vi "BMME385Project2_AmeenZafiruddin.vi"() -> ()   [LabVIEW 2022 SP3]
doc: "Read one the value of one analog channel from a LINX device."
uses:
  <vilib>/Analysis/3filter.llb/Filter Passband Type.ctl
  <vilib>/MakerHub/LINX/Public/Peripherals/Analog/Analog Read 1 Chan.vi
  <vilib>/MakerHub/LINX/Public/Peripherals/Digital/Digital Write N Chans.vi
  <vilib>/MakerHub/LINX/Public/Peripherals/Analog/Analog Read N Chans.vi
  <vilib>/MakerHub/LINX/Private/Local IO/LinxDigitalWrite.vi
  <vilib>/MakerHub/LINX/Public/Utilities/Check Channel.vi
  <vilib>/MakerHub/LINX/Private/Local IO/LinxAnalogRead.vi
  <vilib>/MakerHub/LINX/Private/Utilties/Generate Error.vi
  <vilib>/MakerHub/LINX/LMH-LINX.lvlib
  <vilib>/ptbypt/NI_PtbyPt.lvlib
  <vilib>/Analysis/NI_AAL_SigProc.lvlib
  <vilib>/Analysis/NI_AALBase.lvlib
panel:
  out "Diastolic Pressure":dbl
  out "Closest D Time":dbl
  out "Closest D Time Index":i32
  out "D Time":dbl
  out "D Location":dbl
  out "Systolic Pressure":dbl
  out "Closest S Time":dbl
  out "Closest S Time Index":i32
  out "S Time":dbl
  out "S Location":dbl
  out "Closest D Peak":dbl
  out "Closest D Peak Index":i32
  out "Closest S Peak":dbl
  out "Closest S Peak Index":i32
  out "Diastolic Peak Amp":dbl
  out "Systolic Peak Amp":dbl
  out "Mean Arterial Pressure (MAP)":dbl
  out "Closest MAP Time":dbl
  out "Closest MAP Index":i32
  out "MAP Time":dbl
  out "MAP Location":dbl
  out "MAP Peak Amp":dbl
  out "Amplitudes (mmHg)":dbl[](array[numeric])
  out "Locations":dbl[](array[numeric])
  in  "Peak Detection Threshold":dbl format="%0.2f"
  out "T Subset":dbl[](array[numeric])
  out "O Subset":dbl[](array[numeric])
  out "Oscillations (Bandpass Data) Subset":cluster{dbl[], dbl[]}[](graph)
  in  "Initialize\nFilter":bool
  in  "Filter Type":T1
  in  "Low Cutoff Frequency (Hz)":dbl=0.125 format="%0.3f"
  in  "High Cutoff Frequency (Hz)":dbl=0.45000000000000007 format="%0.3f"
  out "Oscillations (Bandpass Data) (mmHg)":dbl[](array[numeric])
  in  "Subset Start/Stop":bool
  out "Pressure (Raw Data) Subset":cluster{dbl[], dbl[]}[](graph)
  out "P Subset":dbl[](array[numeric])
  out "Time (s)":dbl[](array[numeric])
  out "Pressure (Raw Data) (mmHg)":dbl[](array[numeric])
  out "Pressure (Raw Data) (mmHg)":dbl(graph)
  in  "Digital Out (Gain)":bool[](array[boolean])
  in  "Digital Out Channels":u8[](array[numeric])=[10, 11, 12, 13]
  in  "Set Gain":bool
  in  "AI Channel":u8
  out "Loop Rate (Hz)":u32
  in  "Stop Button":bool
  out "Oscillations (Bandpass Data) (mmHg)":dbl(graph)
  in  "Serial Port":refnum<visa-resource-name>
  # "LINX Device Settings"
  # "Gain Settings"
  # "Filter Settings"
  # "HOW TO USE\n\n1. Connect appropriate hardware to computer via USB (Arduino + LTC615 + Pressure Transducer + BP Cuff)\n2. Select the COM Port (connected USB port) and Analog Channel (A0 - A1 on Arduino) under LINX Device Settings\n3. Set Gain via binary according to the appropriate digital channels (0001 = 128 Gain provided full range) under Gain Settings\n4. Set Filter to bandpass with a frequency range of 1 to 10 Hz under Filter Settings\n5. Click the Run Arrow\n6. Wrap the BP cuff around the patient and click the Initialize Filter button under Filter Settings\n7. Test to see if the raw and filtered pressure data are reading appropriately relative to the gauge attached to the BP cuff\n8. Pump up the cuff to 160 mmHg and begin to slowly release air\n9. Once the pressure reaches 140 mmHg, click the Subset Start/Stop button with an appropriate Peak Detection Threshold\n10. Continue to allow the air to release. Oscillations should be observed on the bandpass data graphs\n11. Once the pressure reaches 50 mmHg, click the Subset Start/Stop button (at least 10 oscillations should be observed on the bandpass data subset)\n12. Release the remaining air from the cuff and click the Compute (Stop) button once the pressure reaches ~0 mmHg\n13. The Mean Arterial Pressure (MAP) and Systolic & Diastolic Blood Pressures should be displayed"
  # "________________________________________________"
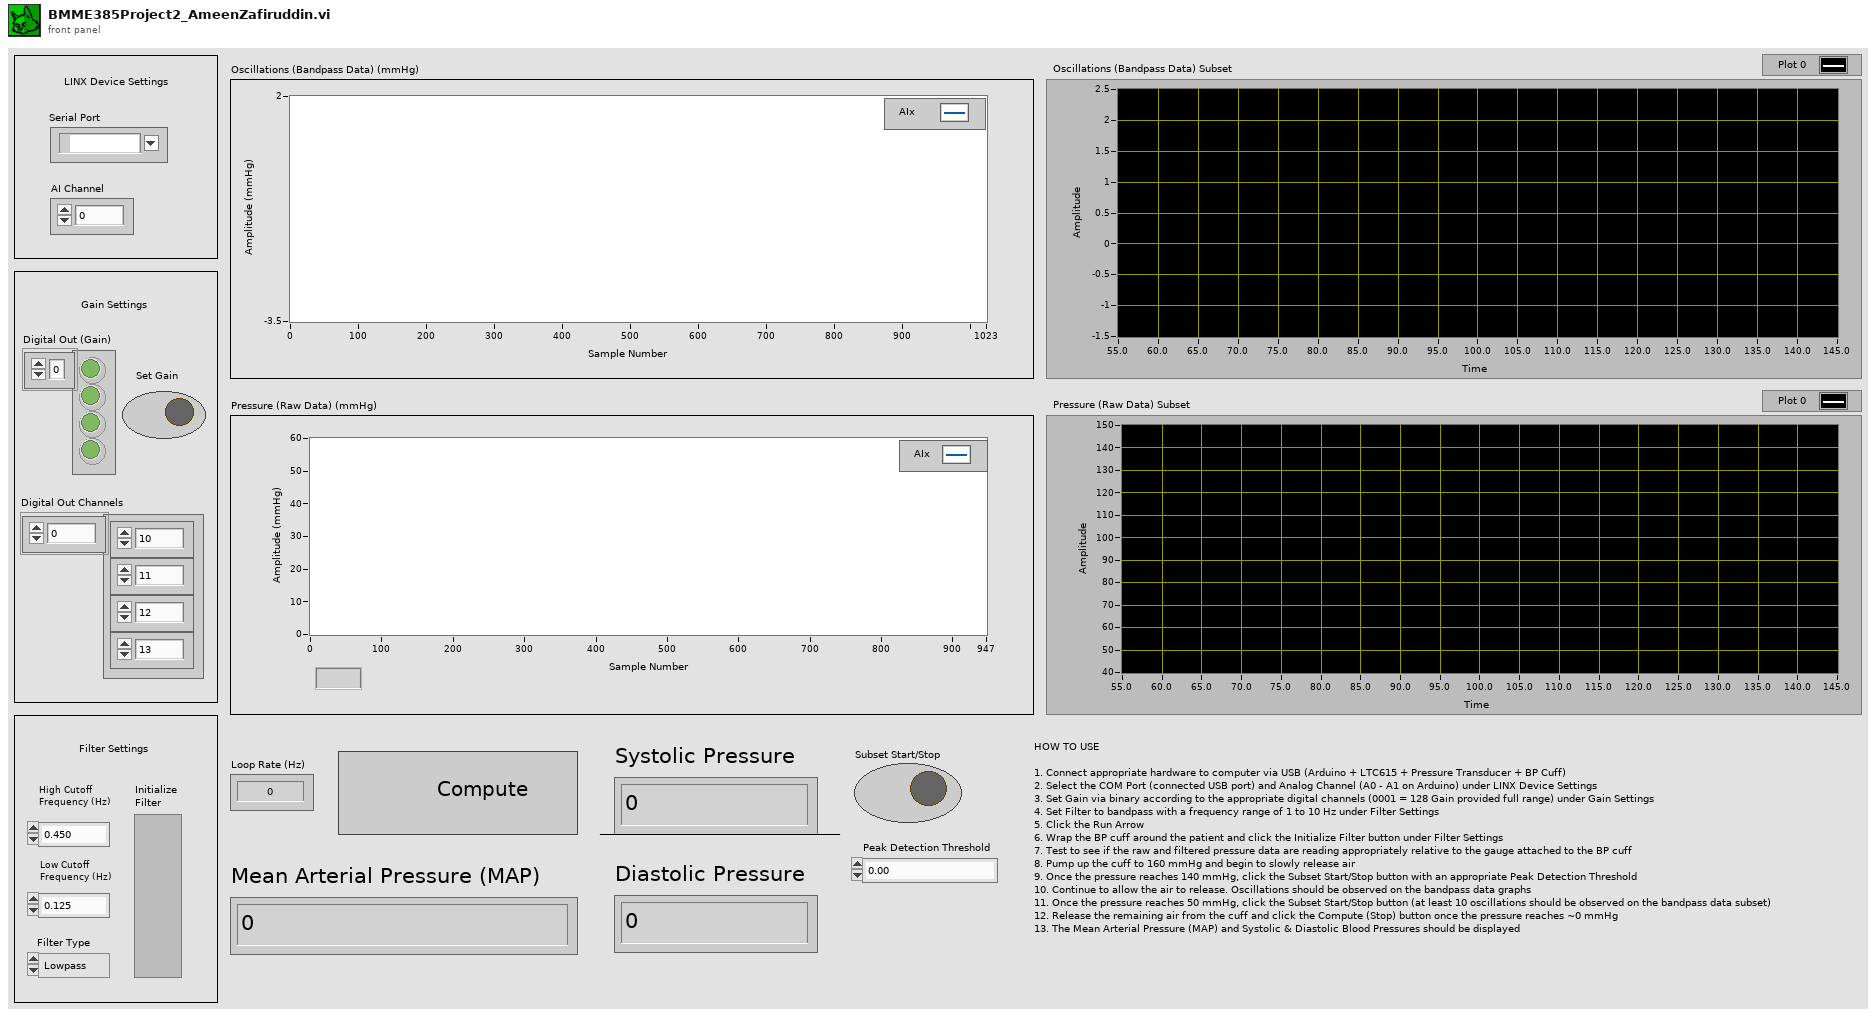
[diagram p1: front panel]
types:
  T1 = typedef "NI_AALBase.lvlib/Filter Passband Type.ctl" = enum32{"Lowpass", "Highpass", "Bandpass", "Bandstop"}
  T2 = typedef "LMH-LINX.lvlib/LINX Ref.ctl" = cluster{"IO":T3, "Interface":T4, "LINX Device Config":T5}
  T3 = typedef "LMH-LINX.lvlib/Platform.ctl" = enum16{"Remote", "Local"}
  T4 = typedef "LMH-LINX.lvlib/Interface.ctl" = enum16{"Serial", "TCP"}
  T5 = typedef "LMH-LINX.lvlib/Device.lvlib/LINX Device Config.ctl" = cluster{"Interface":T4, "COM Port":refnum<visa-resource-name>, "TCP Configuration":T6, "Device Family":u8, "Device ID":u8, "Device Name":string, "TCP Ref":refnum<k5>, "Channels":T7}
  T6 = typedef "LMH-LINX.lvlib/Device.lvlib/TCP Config.ctl" = cluster{"IP Address":string, "Port":u16}
  T7 = typedef "LMH-LINX.lvlib/Channels.ctl" = cluster{"DI":u8[], "DO":u8[], "AI":u8[], "AO":u8[], "PWM":u8[], "QE":u8[], "UART":u8[], "I2C 2":u8[], "SPI":u8[], "CAN":u8[], "Servo":u8[], "AI Ref (V)":dbl, "AI Resolution (Bits)":u8, "AO Ref (V)":dbl, "AO Resolution (Bits)":u8}
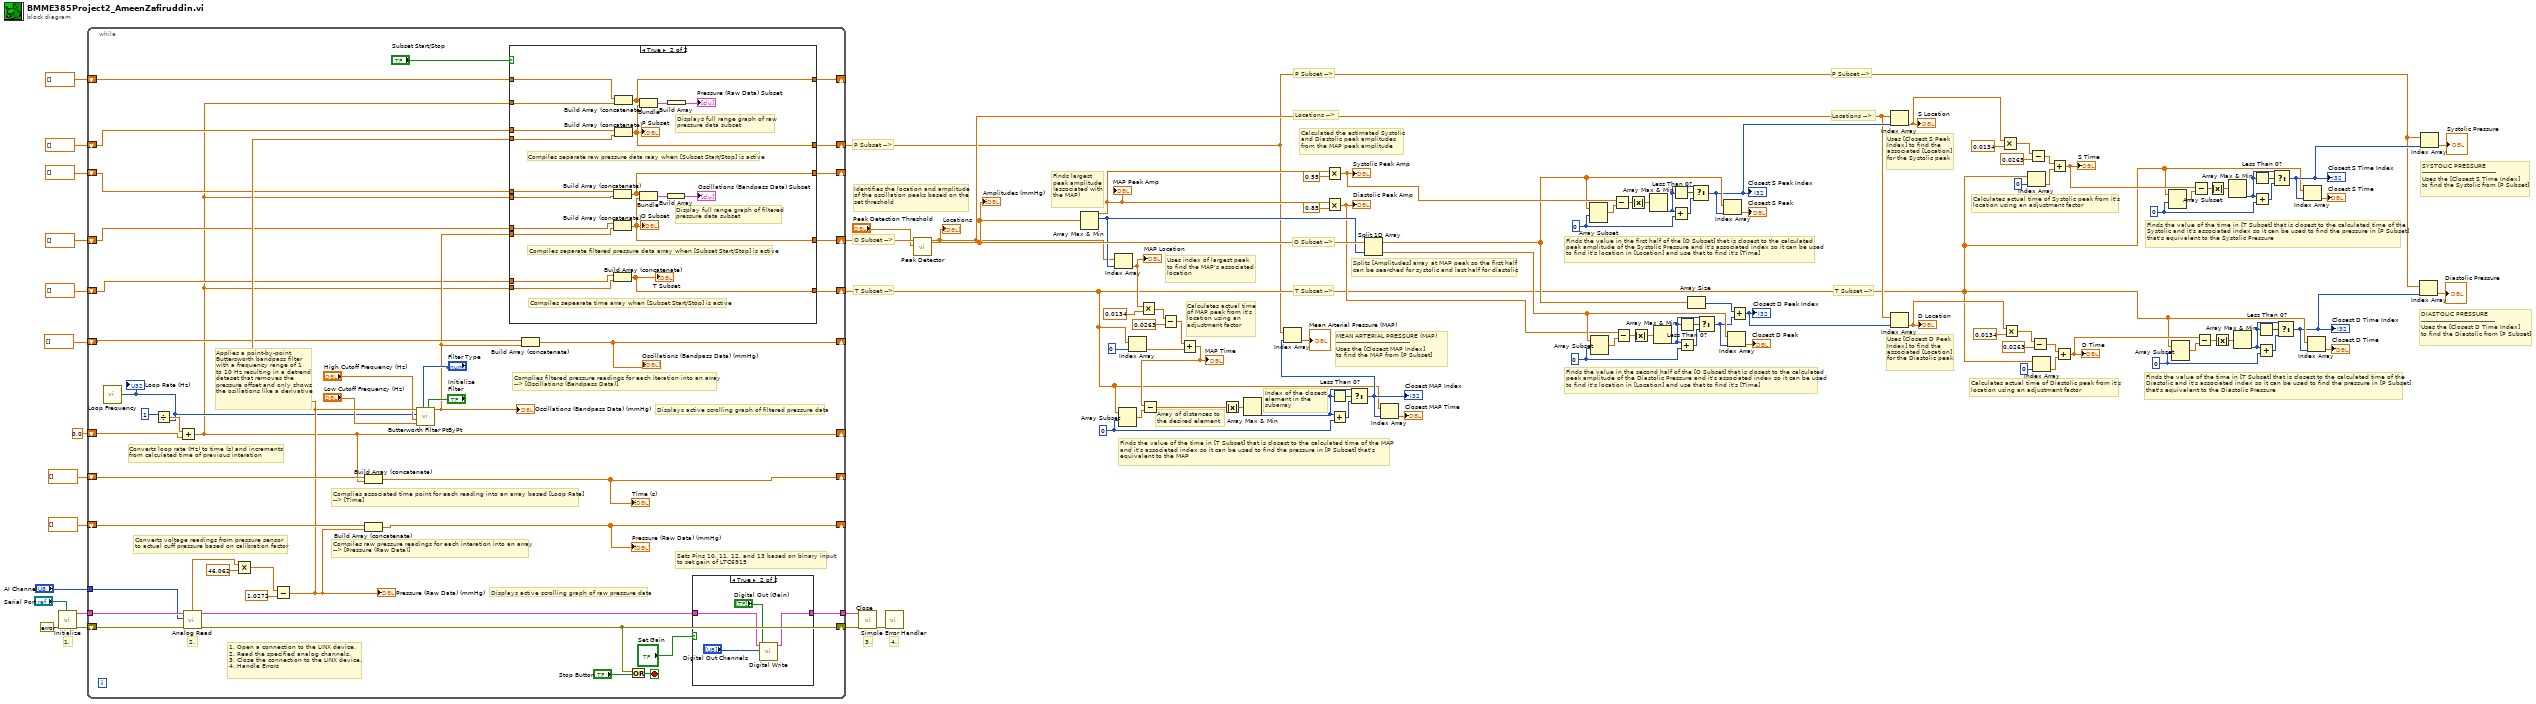
[diagram p0: block diagram]
diagram:
  w6 = 0 ("index")
  w26 = 0 ("index")
  w45 = 0 ("index")
  w46 = 0 ("index")
  w71 = 0 ("index")
  # "DIASTOLIC PRESSURE\n-------------------------------------\nUses the [Closest D Time Index]\nto find the Diastolic from [P Subset]"
  # "SYSTOLIC PRESSURE\n-------------------------------------\nUses the [Closest S Time Index]\nto find the Systolic from [P Subset]"
  # "Finds the value of the time in [T Subset] that is closest to the calculated time of the\nSystolic and it's associated index so it can be used to find the pressure in [P Subset]\nthat's equivalent to the Systolic Pressure"
  # "Finds the value of the time in [T Subset] that is closest to the calculated time of the\nDiastolic and it's associated index so it can be used to find the pressure in [P Subset]\nthat's equivalent to the Diastolic Pressure"
  # "Calculates actual time of Systolic peak from it's\nlocation using an adjustment factor"
  # "Calculates actual time of Diastolic peak from it's\nlocation using an adjustment factor"
  # "Uses [Closest D Peak\nIndex] to find the\nassociated [Location]\nfor the Diastolic peak"
  # "Uses [Closest S Peak\nIndex] to find the\nassociated [Location]\nfor the Systolic peak"
  # "P Subset -->"
  # "Locations -->"
  # "T Subset -->"
  # "Finds the value in the first half of the [O Subset] that is closest to the calculated\npeak amplitude of the Systolic Pressure and it's associated index so it can be used\nto find it's location in [Location] and use that to find it's [Time]"
  # "Finds the value in the second half of the [O Subset] that is closest to the calculated\npeak amplitude of the Diastolic Pressure and it's associated index so it can be used\nto find it's location in [Location] and use that to find it's [Time]"
  # "Splits [Amplitudes] array at MAP peak so the first half\ncan be searched for systolic and last half for diastolic"
  # "Locations -->"
  # "Calculated the estimated Systolic\nand Diastolic peak amplitudes\nfrom the MAP peak amplitude"
  # "P Subset -->"
  # "O Subset -->"
  # "T Subset -->"
  # "MEAN ARTERIAL PRESSURE (MAP)\n-------------------------------------\nUses the [Closest MAP Index]\nto find the MAP from [P Subset]"
  # "Finds the value of the time in [T Subset] that is closest to the calculated time of the MAP\nand it's associated index so it can be used to find the pressure in [P Subset] that's\nequivalent to the MAP"
  # "P Subset -->"
  # "O Subset -->"
  # "T Subset -->"
  # "Calculates actual time\nof MAP peak from it's\nlocation using an\nadjustment factor"
  # "Uses index of largest peak\nto find the MAP's associated\nlocation"
  # "Finds largest\npeak amplitude\n(associated with\nthe MAP)"
  # "Identifies the location and amplitude\nof the oscillation peaks based on the\nset threshold"
  # "Index of the closest element in the subarray"
  # "Array of distances to the desired element"
  # "4."
  # "3."
  # "1."
  n1 = call <vilib>:"Initialize.vi"("Serial Port"="Serial Port", "Error In"=errorcluster {"status"=FALSE, "code"=0, "source"=""}) -> ("Error Out"=w104:errorcluster, "LINX Resource"=w105:T2)  [unwired: 7 in, 1 out]
  n2 = while {
    tunnel: w105 -> [w146]
    tunnel: [w139] -> w103
    shift-right: [w142] -> w102
    shift-left: w104 -> [w145]
    tunnel: "AI Channel" -> [w141]
    shift-right: [w128] -> _
    shift-left: dbl[] [] -> [w133]
    shift-right: [w106] -> _
    shift-left: 0.0 -> [w130]
    shift-right: [w127] -> _
    shift-left: dbl[] [] -> [w129]
    shift-right: [w125] -> _
    shift-left: dbl[] [] -> [w124]
    shift-right: [w123] -> w2
    shift-left: dbl[] [] -> [w122]
    shift-right: [w119] -> _
    shift-left: dbl[] [] -> [w120]
    shift-right: [w113] -> _
    shift-left: dbl[] [] -> [w112]
    shift-right: [w111] -> w88
    shift-left: dbl[] [] -> [w110]
    shift-right: [w108] -> w4
    shift-left: dbl[] [] -> [w107]
    stop <- w144 stop-if-true
    # "1. Open a connection to the LINX device.\n2. Read the specified analog channels.\n3. Close the connection to the LINX device.\n4. Handle Errors"
    # "Complies filtered pressure readings for each iteration into an array\n--> [Oscillations (Bandpass Data)]"
    # "Displays active scrolling graph of filtered pressure data"
    # "Applies a point-by-point\nButtersworth bandpass filter\nwith a frequency range of 1\nto 10 Hz resulting in a detrend\ndataset that removes the\npressure offset and only shows\nthe osillations like a derivative"
    # "Converts loop rate (Hz) to time (s) and increments\nfrom calculated time of previous interation"
    # "Displays active scrolling graph of raw pressure data"
    # "Complies associated time point for each reading into an array based [Loop Rate]\n--> [Time]"
    # "Compiles raw pressure readings for each interation into an array\n--> [Pressure (Raw Data)]"
    # "Converts voltage readings from pressure sensor\nto actual cuff pressure based on calibration factor"
    # "Sets Pins 10, 11, 12, and 13 based on binary input\nto set gain of LTC6915"
    # "2."
    n3 = call <vilib>:"Loop Frequency.vi"() -> ("Loop Rate (Hz)"=w114:u32)
    "Loop Rate (Hz)" <- w114
    n4 = Divide(x=u32 1, y=w114) -> (x/y=w131:dbl)
    n5 = Add(x=w131, y=w130) -> (x+y=w106:dbl)
    n6 = call-poly <vilib>:"Analog Read.vi"("Error In"=w145, "Analog Channel"=w141, "LINX Resource"=w146) -> ("Error Out"=w142:errorcluster, "Voltage"=w137:dbl, "LINX Resource"=w140:T2)  [unwired: 5 in, 1 out]
    n7 = Multiply(x=w137, y=46.062) -> (x*y=w134:dbl)
    n8 = Subtract(x=w134, y=1.0272) -> (x-y=w121:dbl)
    "Pressure (Raw Data) (mmHg)" <- w121
    n9 = Build Array (concatenate)(w133, w121) -> (w128:dbl[])
    "Pressure (Raw Data) (mmHg)" <- w128
    n10 = Build Array (concatenate)(w129, w106) -> (w127:dbl[])
    "Time (s)" <- w127
    n11 = call <vilib>:"Butterworth Filter PtByPt.vi"("initialize"="Initialize\nFilter", "filter type"="Filter Type", "low cutoff freq: fl"="Low Cutoff Frequency (Hz)", "high cutoff freq: fh"="High Cutoff Frequency (Hz)", "sampling freq: fs"=w114, "x"=w121) -> ("Filtered x"=w109:dbl)  [unwired: 3 in, 1 out]
    "Oscillations (Bandpass Data) (mmHg)" <- w109
    n12 = case shown="True" "Subset Start/Stop" {
      tunnel: w124 -> [w151 w170]
      tunnel: [w151 w166] -> w125
      tunnel: w106 -> [_ w169]
      tunnel: w122 -> [w150 w168]
      tunnel: w121 -> [_ w167]
      tunnel: [w150 w165] -> w123
      tunnel: [w149 w160] -> w113
      tunnel: w112 -> [w149 w159]
      tunnel: w106 -> [_ w158]
      tunnel: [w148 w157] -> w111
      tunnel: w110 -> [w148 w156]
      tunnel: w109 -> [_ w155]
      tunnel: [w147 w154] -> w108
      tunnel: w107 -> [w147 w153]
      tunnel: w106 -> [_ w152]
      frame False {
      }
      frame True {
        # "Displays full range graph of raw\npressure data subset"
        # "Display full range graph of filtered\npressure data subset"
        # "Compiles separate raw pressure data raay when [Subset Start/Stop] is active"
        # "Compiles separate filtered pressure data array when [Subset Start/Stop] is active"
        # "Compiles sepearate time array when [Subset Start/Stop] is active"
        n13 = Build Array (concatenate)(w159, w158) -> (w160:dbl[])
        n14 = Build Array (concatenate)(w156, w155) -> (w157:dbl[])
        "O Subset" <- w157
        n15 = Build Array (concatenate)(w153, w152) -> (w154:dbl[])
        "T Subset" <- w154
        n16 = Build Array (concatenate)(w170, w169) -> (w166:dbl[])
        n17 = Build Array (concatenate)(w168, w167) -> (w165:dbl[])
        "P Subset" <- w165
        n18 = Bundle(w160, w157) -> (w162:cluster{dbl[], dbl[]})  [unwired: 1 in]
        n19 = Bundle(w166, w165) -> (w164:cluster{dbl[], dbl[]})  [unwired: 1 in]
        n20 = Build Array(w162) -> (→"Oscillations (Bandpass Data) Subset":cluster{dbl[], dbl[]}[])
        n21 = Build Array(w164) -> (→"Pressure (Raw Data) Subset":cluster{dbl[], dbl[]}[])
      }
    }
    n22 = Build Array (concatenate)(w120, w109) -> (w119:dbl[])
    "Oscillations (Bandpass Data) (mmHg)" <- w119
    n23 = Or(x=w142, y="Stop Button") -> (x .or. y?=w144:bool)
    n24 = case shown="True" "Set Gain" {
      tunnel: w140 -> [w171 w175]
      tunnel: [w171 w174] -> w139
      frame False {
      }
      frame True {
        n25 = call-poly <vilib>:"Digital Write.vi"("Values"="Digital Out (Gain)", "DO Channels"="Digital Out Channels", "LINX Resource"=w175) -> ("LINX Resource"=w174:T2)  [unwired: 7 in, 1 out]
      }
    }
  }
  n26 = call <vilib>:"Close.vi"("Error In"=w102, "LINX Resource"=w103) -> ("Error Out"=w100:errorcluster)  [unwired: 9 in]
  n27 = call <vilib>:"Simple Error Handler.vi"("error in (no error)"=w100) -> ()  [unwired: 4 in, 5 out]
  n28 = call <vilib>:"Peak Detector.vi"("threshold"="Peak Detection Threshold", "X"=w88) -> ("Amplitudes"=w65:dbl[], "Locations"=w16:dbl[])  [unwired: 5 in, 3 out]
  "Locations" <- w16
  "Amplitudes (mmHg)" <- w65
  n29 = Array Max & Min(array=w65) -> (max value=w68:dbl, max index (indices)=w64:i32)  [unwired: 2 out]
  "MAP Peak Amp" <- w68
  n30 = Index Array(array=w16, index=w64) -> (element=w86:dbl)
  "MAP Location" <- w86
  n31 = Array Subset(array=w4, index=w71) -> (w73:dbl[])  [unwired: 1 in]
  n32 = Index Array(array=w4, index=0) -> (element=w80:dbl)
  n33 = Multiply(x=w86, y=0.0134) -> (x*y=w84:dbl)
  n34 = Subtract(x=w84, y=0.0263) -> (x-y=w81:dbl)
  n35 = Add(x=w81, y=w80) -> (x+y=w72:dbl)
  "MAP Time" <- w72
  n36 = Subtract(x=w72, y=w73) -> (x-y=w79:dbl[])
  n37 = Absolute Value(x=w79) -> (abs(x)=w77:dbl[])
  n38 = Array Max & Min(array=w77) -> (min index (indices)=w75:i32)  [unwired: 3 out]
  n39 = Multiply(x=w68, y=0.55) -> (x*y=w48:dbl)
  "Systolic Peak Amp" <- w48
  n40 = Multiply(x=w68, y=0.85) -> (x*y=w47:dbl)
  "Diastolic Peak Amp" <- w47
  n41 = Less Than 0?(x=w75) -> (x < 0?=w76:bool)
  n42 = Add(x=w75, y=w71) -> (x+y=w74:i32)
  n43 = Select(t=w75, s=w76, f=w74) -> (s? t:f=w70:i32)
  "Closest MAP Index" <- w70
  n44 = Index Array(array=w2, index=w70) -> (element=→"Mean Arterial Pressure (MAP)":dbl)
  n45 = Split 1D Array(array=w65, index=w64) -> (first subarray=w44:dbl[], second subarray=w49:dbl[])
  n46 = Index Array(array=w4, index=w70) -> (element=→"Closest MAP Time":dbl)
  n47 = Array Subset(array=w44, index=w45) -> (w57:dbl[])  [unwired: 1 in]
  n48 = Array Subset(array=w49, index=w46) -> (w50:dbl[])  [unwired: 1 in]
  n49 = Subtract(x=w48, y=w57) -> (x-y=w63:dbl[])
  n50 = Subtract(x=w47, y=w50) -> (x-y=w56:dbl[])
  n51 = Absolute Value(x=w63) -> (abs(x)=w61:dbl[])
  n52 = Absolute Value(x=w56) -> (abs(x)=w54:dbl[])
  n53 = Array Max & Min(array=w61) -> (min index (indices)=w59:i32)  [unwired: 3 out]
  n54 = Array Max & Min(array=w54) -> (min index (indices)=w52:i32)  [unwired: 3 out]
  n55 = Less Than 0?(x=w59) -> (x < 0?=w60:bool)
  n56 = Add(x=w59, y=w45) -> (x+y=w58:i32)
  n57 = Less Than 0?(x=w52) -> (x < 0?=w53:bool)
  n58 = Add(x=w52, y=w46) -> (x+y=w51:i32)
  n59 = Array Size(array=w44) -> (size(s)=w43:i32)
  n60 = Select(t=w59, s=w60, f=w58) -> (s? t:f=w41:i32)
  "Closest S Peak Index" <- w41
  n61 = Select(t=w52, s=w53, f=w51) -> (s? t:f=w42:i32)
  n62 = Index Array(array=w44, index=w41) -> (element=→"Closest S Peak":dbl)
  n63 = Index Array(array=w49, index=w42) -> (element=→"Closest D Peak":dbl)
  n64 = Add(x=w43, y=w42) -> (x+y=w17:i32)
  "Closest D Peak Index" <- w17
  n65 = Index Array(array=w16, index=w41) -> (element=w37:dbl)
  "S Location" <- w37
  n66 = Index Array(array=w16, index=w17) -> (element=w19:dbl)
  "D Location" <- w19
  n67 = Multiply(x=w37, y=0.0134) -> (x*y=w39:dbl)
  n68 = Multiply(x=w19, y=0.0134) -> (x*y=w21:dbl)
  n69 = Index Array(array=w4, index=0) -> (element=w34:dbl)
  n70 = Subtract(x=w39, y=0.0263) -> (x-y=w36:dbl)
  n71 = Subtract(x=w21, y=0.0263) -> (x-y=w18:dbl)
  n72 = Index Array(array=w4, index=0) -> (element=w14:dbl)
  n73 = Add(x=w36, y=w34) -> (x+y=w25:dbl)
  "S Time" <- w25
  n74 = Add(x=w18, y=w14) -> (x+y=w5:dbl)
  "D Time" <- w5
  n75 = Array Subset(array=w4, index=w26) -> (w27:dbl[])  [unwired: 1 in]
  n76 = Array Subset(array=w4, index=w6) -> (w7:dbl[])  [unwired: 1 in]
  n77 = Subtract(x=w25, y=w27) -> (x-y=w33:dbl[])
  n78 = Subtract(x=w5, y=w7) -> (x-y=w13:dbl[])
  n79 = Absolute Value(x=w33) -> (abs(x)=w31:dbl[])
  n80 = Absolute Value(x=w13) -> (abs(x)=w11:dbl[])
  n81 = Array Max & Min(array=w31) -> (min index (indices)=w29:i32)  [unwired: 3 out]
  n82 = Array Max & Min(array=w11) -> (min index (indices)=w9:i32)  [unwired: 3 out]
  n83 = Less Than 0?(x=w29) -> (x < 0?=w30:bool)
  n84 = Add(x=w29, y=w26) -> (x+y=w28:i32)
  n85 = Less Than 0?(x=w9) -> (x < 0?=w10:bool)
  n86 = Add(x=w9, y=w6) -> (x+y=w8:i32)
  n87 = Select(t=w29, s=w30, f=w28) -> (s? t:f=w24:i32)
  "Closest S Time Index" <- w24
  n88 = Select(t=w9, s=w10, f=w8) -> (s? t:f=w3:i32)
  "Closest D Time Index" <- w3
  n89 = Index Array(array=w4, index=w24) -> (element=→"Closest S Time":dbl)
  n90 = Index Array(array=w4, index=w3) -> (element=→"Closest D Time":dbl)
  n91 = Index Array(array=w2, index=w3) -> (element=→"Diastolic Pressure":dbl)
  n92 = Index Array(array=w2, index=w24) -> (element=→"Systolic Pressure":dbl)
